vi "Configure Samples per Scan.vi"(8 "error in (no error)":errorcluster, 10 "Select Samples Per Scan":T1(ring), 11 "PF_API in":refnum<class "PF_API.lvclass">) -> (0 "error out":errorcluster, 3 "PF_API out":refnum<class "PF_API.lvclass">)   [LabVIEW 2019, in "PF_API.lvclass"]
doc: "Defines the samples per scan and scan frequency."
uses:
  PF_API.lvclass
  PF_API.lvclass/PF_API.ctl
  <vilib>/httpClient/POSTBuffer.vi
  <vilib>/httpClient/LabVIEWHTTPClient.lvlib
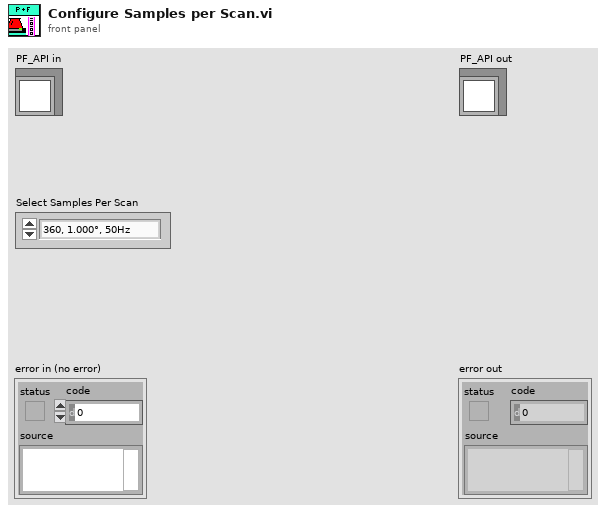
[diagram p1: front panel]
types:
  T1 = enum16{"360, 1.000°, 50Hz", "720, 0.500°, 50Hz", "1440, 0.250°, 50Hz", "360, 1.000°, 35Hz", "720, 0.500°, 35Hz", "1440, 0.250°, 35Hz", "360, 1.000°, 10Hz", "720, 0.500°, 10Hz", "1440, 0.250°, 10Hz"}
  T2 = typedef "LabVIEWHTTPClient.lvlib/ClientHandle.ctl" = refnum<k1>
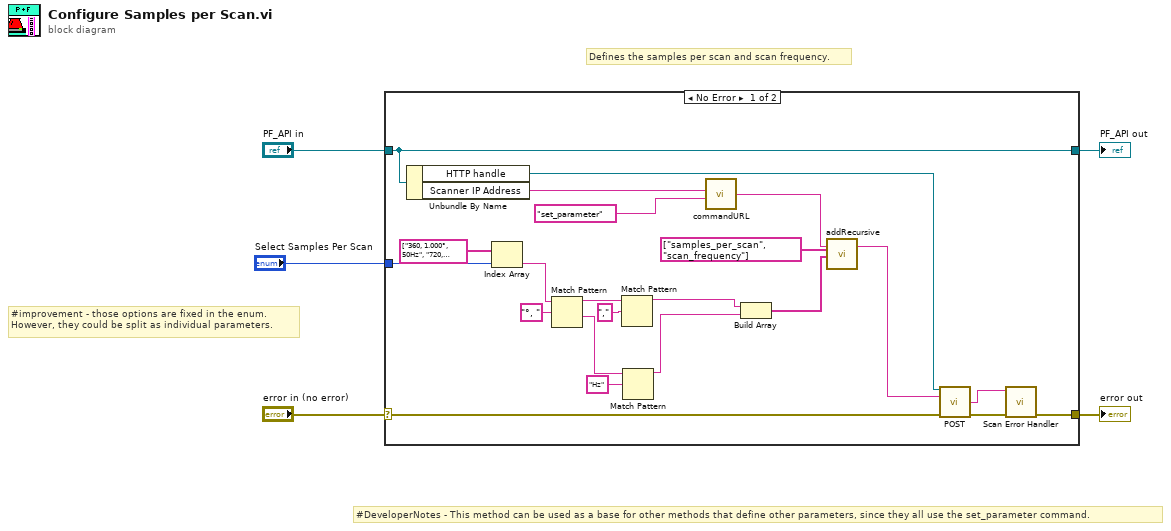
[diagram p0: block diagram]
diagram:
  # "#DeveloperNotes - This method can be used as a base for other methods that define other parameters, since they all use the set_parameter command."
  # "Defines the samples per scan and scan frequency."
  # "#improvement - those options are fixed in the enum.\nHowever, they could be split as individual parameters."
  n1 = case shown="No Error" "error in (no error)" {
    selector: "error in (no error)" -> [w27 w29]
    tunnel: [w9 w29] -> w4
    tunnel: [w24 w28] -> w2
    tunnel: "PF_API in" -> [w24 w28]
    tunnel: "Select Samples Per Scan" -> [w25 _]
    frame No Error {
      n2 = Unbundle By Name(w24) -> ("HTTP handle"=w6:T2, "Scanner IP Address"=w23:string)
      n3 = Index Array(array=string[] ["360, 1.000°, 50Hz", "720, 0.500°, 50Hz", "1440, 0.250°, 50Hz", "360, 1.000°, 35Hz", "720, 0.500°, 35Hz", "1440, 0.250°, 35Hz", "360, 1.000°, 10Hz", "720, 0.500°, 10Hz", "1440, 0.250°, 10Hz", "480, 0.250°, 50Hz"] ("Strings []"), index=w25) -> (element=w12:string)
      n4 = Match Pattern(string=w12, regular expression="°, ") -> (before substring=w19:string, after substring=w16:string)  [unwired: 1 in, 2 out]
      n5 = Match Pattern(string=w19, regular expression=",") -> (before substring=w14:string)  [unwired: 1 in, 3 out]
      n6 = Match Pattern(string=w16, regular expression="Hz") -> (before substring=w13:string)  [unwired: 1 in, 3 out]
      n7 = call "commandURL.vi"("Command String"="set_parameter", "Scanner IP Address"=w23) -> ("Command URL"=w20:string)  [unwired: 4 in]
      n8 = Build Array(w14, w13) -> (w11:string[])
      n9 = call "addRecursive.vi"("Command URL in"=w20, "Parameter Key"=string[] ["samples_per_scan", "scan_frequency"] ("string"), "Parameter Value"=w11) -> ("Command URL out"=w7:string)  [unwired: 13 in, 3 out]
      n10 = call-poly <vilib>:"POST.vi"("client handle"=w6, "url"=w7, "error in (no error)"=w27) -> ("body"=w8:string, "error out"=w10:errorcluster)  [unwired: 9 in, 2 out]
      n11 = call "Scan Error Handler.vi"("Error In"=w10, "HTTP Response"=w8) -> ("Error Out"=w9:errorcluster)  [unwired: 9 in]
    }
    frame Error {
    }
  }
  "error out" <- w4
  "PF_API out" <- w2
